vi "TelemetryServer_Connect.vi"(4 "Channel Name":string, 5 "Server Name":string, 6 "error in (no error)":errorcluster) -> (0 "error out":errorcluster, 3 "Channel Id":u32)   [LabVIEW 2009]
uses:
  TelemetryServer_Global.vi
  lib/lvrtc.dll
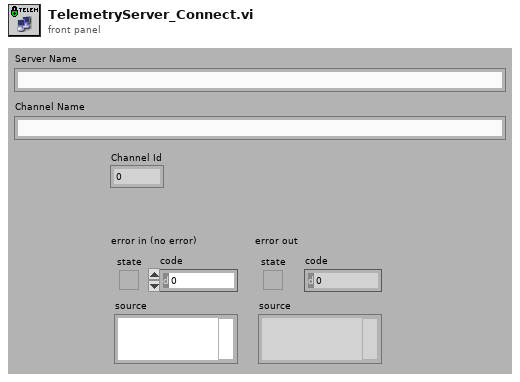
[diagram p1: front panel]
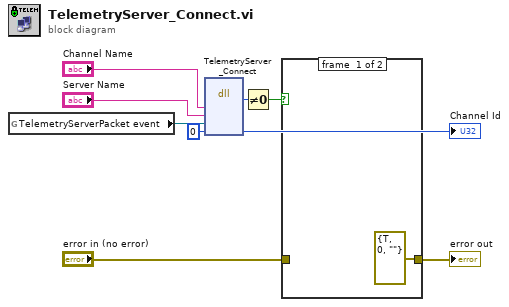
[diagram p0: block diagram]
diagram:
  n1 = global read "TelemetryServer_Global.vi" "TelemetryServerPacket event"() -> (w9:refnum<user-event>)
  n2 = dll-call lib="C:/Ohana/LV2009/OhanaOS-LV81/Instruments/RTC/Api/lib/lvrtc.dll" fn="TelemetryServer_Connect"("channelNameHdl"="Channel Name", "serverNameHdl"="Server Name", "TelemetryServerPacket event"=w9, "id"=u32 0) -> (w4:u32, "id"=→"Channel Id":u32)  [unwired: 6 in, 2 out]
  n3 = Not Equal To 0?(x=w4) -> (x != 0?=w3:bool)
  n4 = case shown="True" w3 {
    tunnel: "error in (no error)" -> [_ w11]
    tunnel: [errorcluster {"status"=TRUE, "code"=0, "source"=""} ("error in (no error)") w11] -> w1
    frame #0 {
    }
    frame #1 {
    }
  }
  "error out" <- w1
